vi "_Validate Ramp Parameter.vi"(5 "error in (no error)":errorcluster) -> (0 "error out":errorcluster, 1 "Steps":i32=1, 3 "Primary Parameter":T1, 4 "Ramp Parameters":T1[](array[typedef]))   [LabVIEW 2012]
uses:
  Type/_Ramp Parameter.ctl
  _Global Configuration.vi
panel:
  # "Gather and validate all ramping parameters and determine the primary ramping channel by choosing the channel with the longest Dwell time.\n\nCalculate the number of ramping steps and use the # of scans and Pause time from the primary ramping parameters."
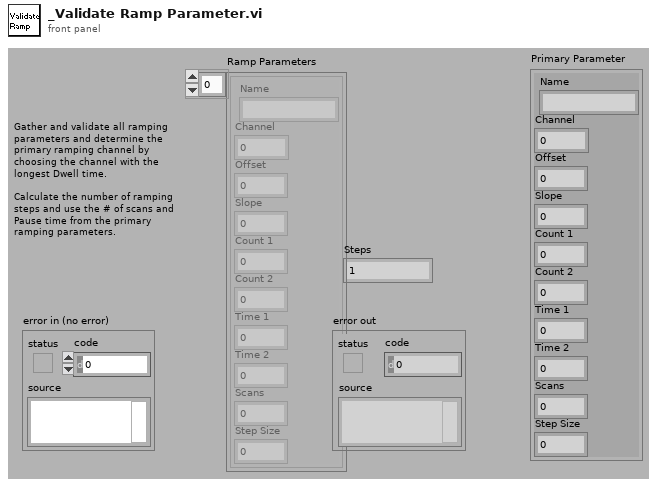
[diagram p1: front panel]
types:
  T1 = typedef "_Ramp Parameter.ctl" = cluster{"Name":string, "Channel":u8, "Offset":dbl, "Slope":dbl, "Count 1":dbl, "Count 2":dbl, "Time 1":dbl, "Time 2":dbl, "Scans":i32, "Step Size":dbl}
  T2 = typedef "_RT Instrument 2.ctl" = cluster{"Table":T3[], "Instrument":string[]}
  T3 = typedef "_RT Configuration 2.ctl" = cluster{"Name":string, "Ch#":u8, "Min":dbl, "Max":dbl, "Def+":dbl, "Def-":dbl, "Offset":dbl, "Slope":dbl, "Type":u8, "Description":string, "SettleT":dbl}
  T4 = typedef "_Lens Property.ctl" = cluster{"Scan Type":u8, "Scans":i32, "Time 1":dbl, "Time 2":dbl, "Value 1":dbl, "Value 2":dbl, "Step Size":dbl}
  T5 = typedef "_Mass Range Property.ctl" = cluster{"Start":dbl, "Stop":dbl, "Step Size":dbl, "Steps":i32, "Dwell":dbl, "Parameters":T6[], "Res":T7}
  T6 = typedef "_Mass Range Parameters.ctl" = cluster{"Name":string, "Ch#":u8, "StartV":dbl, "StopV":dbl, "StepV":dbl, "Index":u8}
  T7 = typedef "_RT Res Type.ctl" = u16
  T8 = typedef "_Run Mode.ctl" = enum16{"MRM (Q1/Q2)", "Q1 Scan", "Q1 SRM", "Q2 Scan", "Q2 SRM", "Product Scan", "Precursor Scan", "Neutral Loss", "Neutral Gain"}
  T9 = cluster{"Lenses":T4[], "Mass Ranges":T5[], "Acquire":bool, "MCA":bool, "Q1DC EN":bool, "Q1 POL":bool, "Q3 POL":bool, "Q1 RF  EN":bool, "Averaging":bool, "Log Scale":bool, "CPS":bool, "Unit":bool, "Data Path":path, "Run Mode":T8, "Fixed Mass (amu)":dbl, "Q3DC EN":bool, "Q3 RF  EN":bool, "Negative":bool}
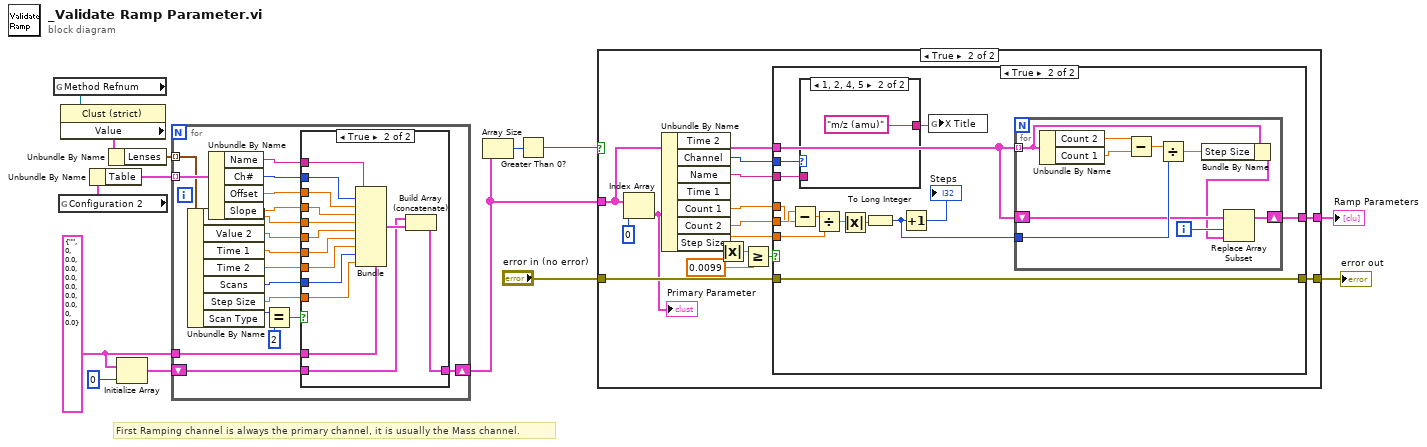
[diagram p0: block diagram]
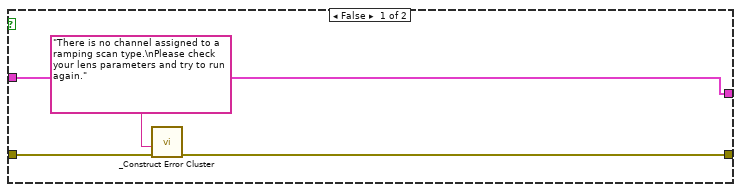
[diagram p2: hidden frame]
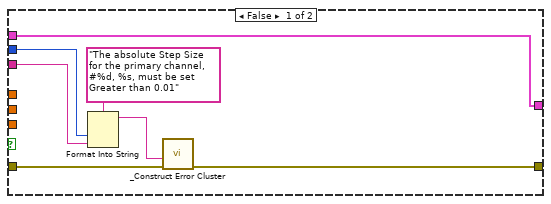
[diagram p3: hidden frame]
diagram:
  w13 = T1 {"Name"="", "Channel"=0, "Offset"=0.0, "Slope"=0.0, "Count 1"=0.0, "Count 2"=0.0, "Time 1"=0.0, "Time 2"=0.0, "Scans"=0, "Step Size"=0.0} ("Ramp Parameter")
  # "First Ramping channel is always the primary channel, it is usually the Mass channel."
  n1 = global read "_Global Configuration.vi" "Method Refnum"() -> (w3:refnum<vi>)
  n2 = global read "_Global Configuration.vi" "Configuration 2"() -> (w5:T2)
  n3 = property class="Clust (strict)"(reference=w3) -> ("Value"=w2:T9)  [unwired: 1 in, 2 out]
  n4 = Unbundle By Name(w5) -> ("Table"=w4:T3[])
  n5 = Unbundle By Name(w2) -> ("Lenses"=w1:T4[])
  n6 = Initialize Array(w13, 0 ("dimension size")) -> (w14:T1[])
  n7 = for {
    shift-right: [w26] -> w12
    shift-left: w14 -> [w27]
    tunnel: w13 -> [w25]
    tunnel: w4 -> [w24] mode=indexing
    tunnel: w1 -> [w23] mode=indexing
    n8 = Unbundle By Name(w23) -> ("Value 1"=w22:dbl, "Value 2"=w21:dbl, "Time 1"=w20:dbl, "Time 2"=w19:dbl, "Scans"=w18:i32, "Step Size"=w17:dbl, "Scan Type"=w16:u8)
    n9 = Unbundle By Name(w24) -> ("Name"=w31:string, "Ch#"=w30:u8, "Offset"=w29:dbl, "Slope"=w28:dbl)
    n10 = Equal?(x=w16, y=u8 2) -> (x = y?=w32:bool)
    n11 = case shown="True" w32 {
      tunnel: w22 -> [_ w47]
      tunnel: w31 -> [_ w46]
      tunnel: w30 -> [_ w45]
      tunnel: w29 -> [_ w44]
      tunnel: w28 -> [_ w43]
      tunnel: w21 -> [_ w42]
      tunnel: w20 -> [_ w35]
      tunnel: w19 -> [_ w34]
      tunnel: w18 -> [_ w41]
      tunnel: w17 -> [_ w40]
      tunnel: w27 -> [w33 w38]
      tunnel: [w33 w36] -> w26
      tunnel: w25 -> [_ w37]
      frame False {
      }
      frame True {
        n12 = Bundle(cluster=w37, "Name"=w46, "Channel"=w45, "Offset"=w44, "Slope"=w43, "Count 1"=w47, "Count 2"=w42, "Time 1"=w35, "Time 2"=w34, "Scans"=w41, "Step Size"=w40) -> (w39:T1)
        n13 = Build Array (concatenate)(w38, w39) -> (w36:T1[])
      }
    }
  }
  n14 = Array Size(array=w12) -> (size(s)=w11:i32)
  n15 = Greater Than 0?(x=w11) -> (x > 0?=w10:bool)
  n16 = case shown="True" w10 {
    tunnel: w12 -> [w48 w57]
    tunnel: "error in (no error)" -> [w51 w63]
    tunnel: [w50 w62] -> w8
    tunnel: [w48 w54] -> w6
    frame False {
      n17 = call "_Construct Error Cluster.vi"("error in"=w51, "reason"="There is no channel assigned to a ramping scan type.\nPlease check your lens parameters and try to run again.") -> ("error out"=w50:errorcluster)  [unwired: 2 in, 3 out]
    }
    frame True {
      n18 = Index Array(array=w57, index=0) -> (element=w56:T1)
      "Primary Parameter" <- w56
      n19 = Unbundle By Name(w56) -> ("Channel"=w59:u8, "Name"=w58:string, "Count 1"=w61:dbl, "Count 2"=w60:dbl, "Step Size"=w53:dbl)  [unwired: 2 out]
      n20 = Absolute Value(x=w53) -> (abs(x)=w52:dbl)
      n21 = Greater Or Equal?(x=w52, y=0.0099) -> (x >= y?=w64:bool)
      n22 = case shown="True" w64 {
        tunnel: w63 -> [w72 w85]
        tunnel: [w71 w85] -> w62
        tunnel: w61 -> [_ w76]
        tunnel: w60 -> [_ w77]
        tunnel: w53 -> [_ w83]
        tunnel: w59 -> [w69 w73]
        tunnel: w58 -> [w68 w80]
        tunnel: w57 -> [w66 w84]
        tunnel: [w66 w79] -> w54
        frame False {
          n23 = Format Into String(format string="The absolute Step Size for the primary channel, #%d, %s, must be set Greater than 0.01", w69, w68) -> (resulting string=w67:string)  [unwired: 2 in, 1 out]
          n24 = call "_Construct Error Cluster.vi"("error in"=w72, "reason"=w67) -> ("error out"=w71:errorcluster)  [unwired: 2 in, 3 out]
        }
        frame True {
          n25 = Subtract(x=w77, y=w76) -> (x-y=w78:dbl)
          n26 = case shown="1, 2, 4, 5" w73 {
            tunnel: [w87 "m/z (amu)" ("y")] -> w81
            tunnel: w80 -> [w87 _]
            frame 0, Default {
            }
            frame 1, 2, 4, 5 {
            }
          }
          n27 = Divide(x=w78, y=w83) -> (x/y=w75:dbl)
          n28 = Absolute Value(x=w75) -> (abs(x)=w74:dbl)
          n29 = To Long Integer(number=w74) -> (32bit integer=w82:i32)
          n30 = Increment(x=w82) -> (x+1=→"Steps":i32)
          n31 = global write "_Global Configuration.vi" "X Title"(w81) -> ()
          n32 = for {
            tunnel: w84 -> [w95] mode=indexing
            shift-right: [w91] -> w79
            shift-left: w84 -> [w93]
            tunnel: w82 -> [w96]
            i -> [w92]
            n33 = Unbundle By Name(w95) -> ("Count 2"=w98:dbl, "Count 1"=w97:dbl)
            n34 = Subtract(x=w98, y=w97) -> (x-y=w89:dbl)
            n35 = Divide(x=w89, y=w96) -> (x/y=w94:dbl)
            n36 = Bundle By Name(cluster=w95, "Step Size"=w94) -> (w90:T1)
            n37 = Replace Array Subset(array=w93, new element=w90, index=w92) -> (w91:T1[])
          }
        }
      }
    }
  }
  "error out" <- w8
  "Ramp Parameters" <- w6
